vi "Manage sensor alert.vi"(7 "Application path":path, 8 "Error In":errorcluster, 9 "Humidity":dbl, 10 "Temperature":dbl, 11 "MAC address":string) -> (0 "Error Out":errorcluster)   [LabVIEW 2016]
uses:
  <vilib>/Utility/config.llb/Read Key (Boolean).vi
  <vilib>/Utility/config.llb/Read Key (Double).vi
  <vilib>/Utility/config.llb/Read Key (String).vi
  <vilib>/Utility/SMTP/NI_SMTPEmail.lvlib
  <vilib>/Utility/config.llb/NI_LVConfig.lvlib
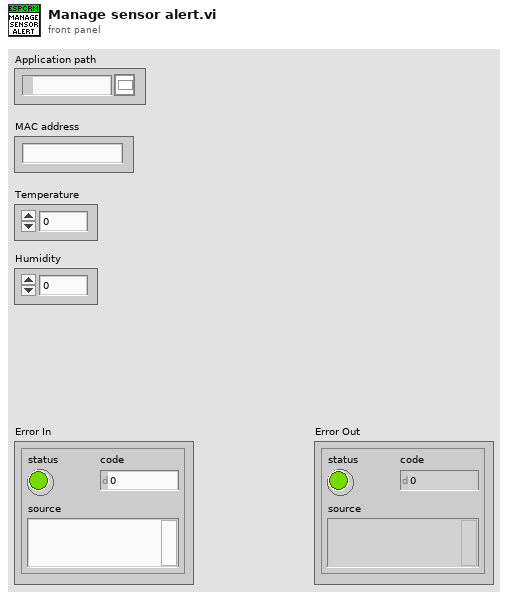
[diagram p1: front panel]
types:
  T1 = typedef "NI_LVConfig.lvlib/Config Data RefNum.ctl" = refnum<k1>
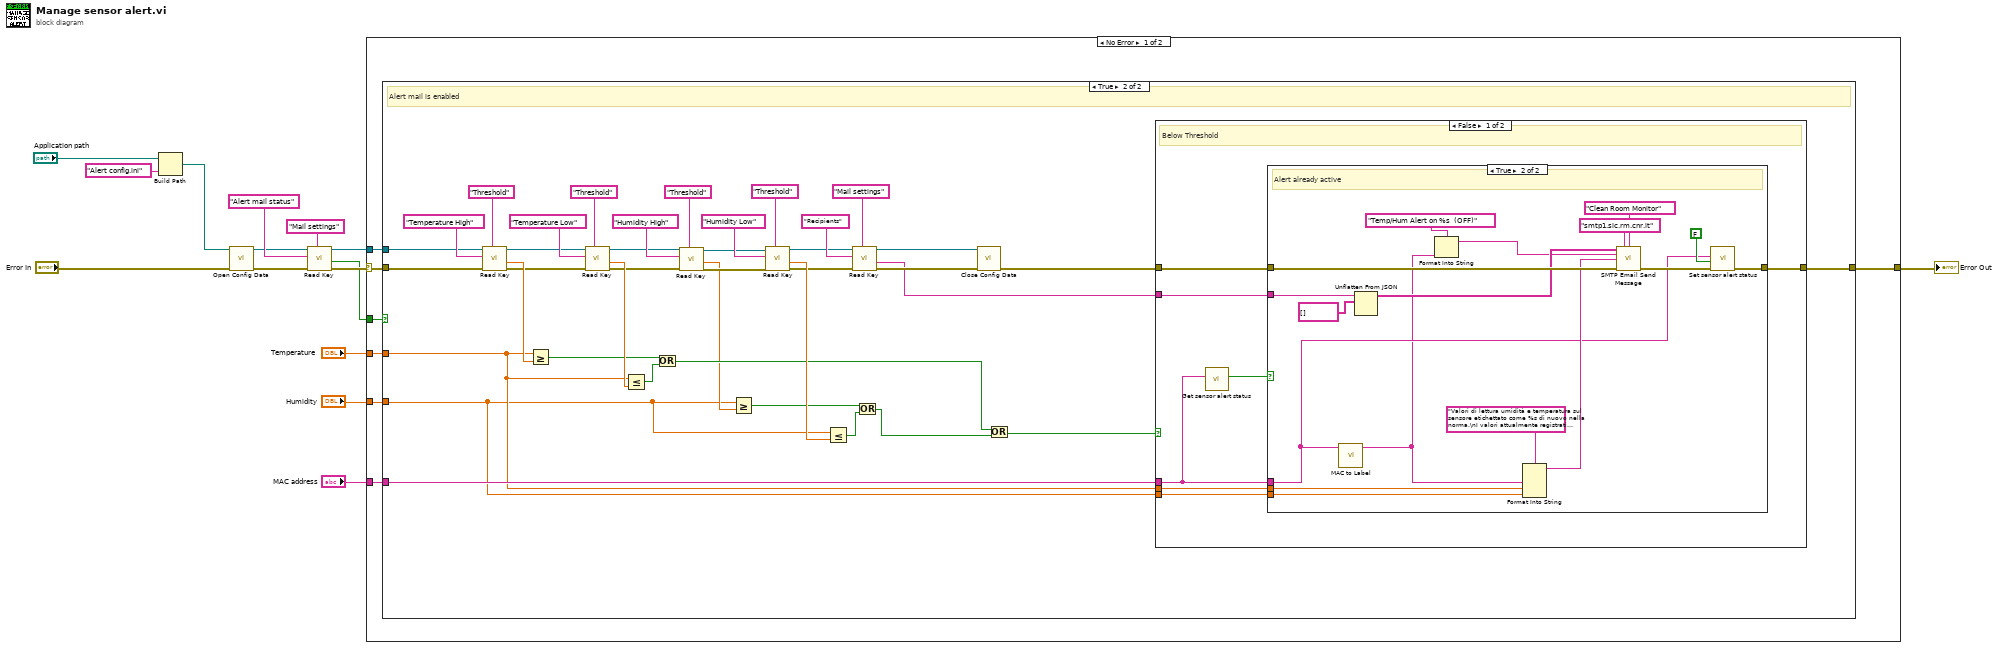
[diagram p0: block diagram]
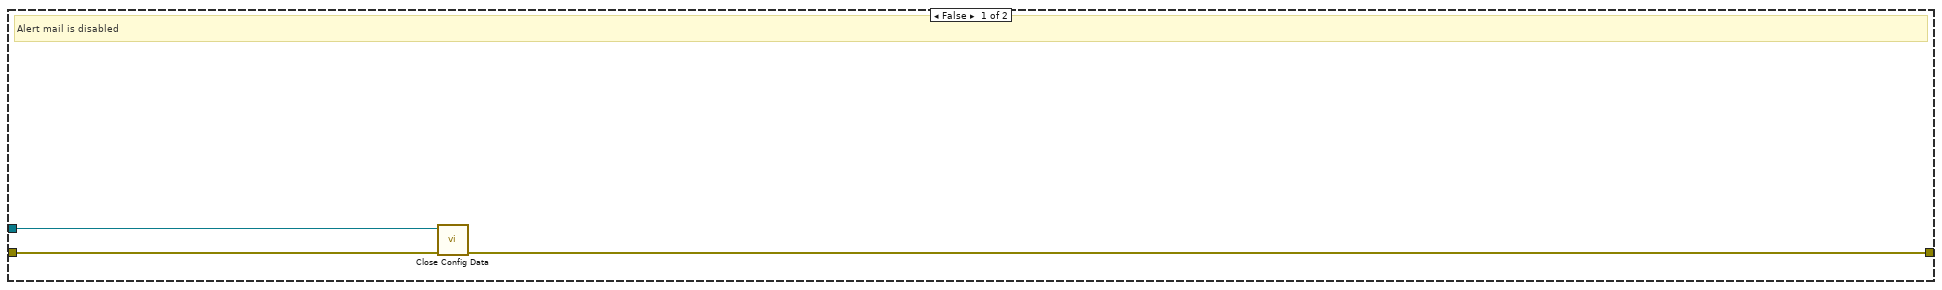
[diagram p2: hidden frame]
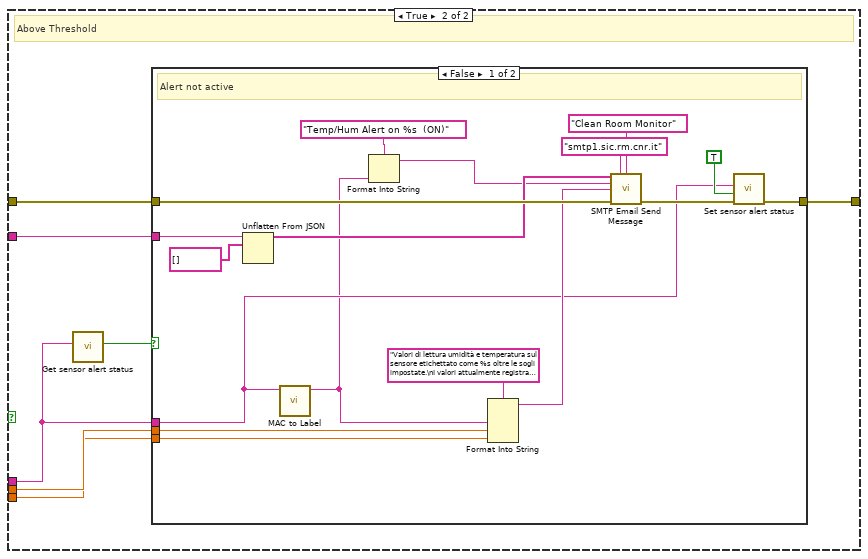
[diagram p4: hidden frame]
diagram:
  n1 = Build Path(base path="Application path", name or relative path="Alert config.ini") -> (appended path=w14:path)
  n2 = call <vilib>:"Open Config Data.vi"("error in (no error)"="Error In", "configuration file path"=w14) -> ("error out"=w9:errorcluster, "refnum"=w10:T1)  [unwired: 7 in, 1 out]
  n3 = call-poly <vilib>:"Read Key.vi"("section"="Mail settings", "error in (no error)"=w9, "key"="Alert mail status", "refnum"=w10) -> ("error out"=w7:errorcluster, "value"=w5:bool, "refnum out"=w8:T1)  [unwired: 4 in, 1 out]
  n4 = case shown="No Error" w7 {
    selector: w7 -> [w21 w115]
    tunnel: [w17 w115] -> w15
    tunnel: w8 -> [w20 _]
    tunnel: w5 -> [w22 _]
    tunnel: "Temperature" -> [w19 _]
    tunnel: "Humidity" -> [w18 _]
    tunnel: "MAC address" -> [w16 _]
    frame No Error {
      n5 = case shown="True" w22 {
        tunnel: w21 -> [w25 w55]
        tunnel: w20 -> [w23 w56]
        tunnel: w19 -> [_ w40]
        tunnel: w18 -> [_ w29]
        tunnel: [w24 w53] -> w17
        tunnel: w16 -> [_ w52]
        frame False {
          # "Alert mail is disabled"
          n6 = call <vilib>:"Close Config Data.vi"("error in (no error)"=w25, "refnum"=w23) -> ("error out"=w24:errorcluster)  [unwired: 8 in, 1 out]
        }
        frame True {
          # "Alert mail is enabled"
          n7 = call-poly <vilib>:"Read Key.vi"("section"="Threshold", "error in (no error)"=w55, "key"="Temperature High", "refnum"=w56) -> ("error out"=w43:errorcluster, "value"=w51:dbl, "refnum out"=w42:T1)  [unwired: 4 in, 1 out]
          n8 = Greater Or Equal?(x=w40, y=w51) -> (x >= y?=w38:bool)
          n9 = call-poly <vilib>:"Read Key.vi"("section"="Threshold", "error in (no error)"=w43, "key"="Temperature Low", "refnum"=w42) -> ("error out"=w33:errorcluster, "value"=w41:dbl, "refnum out"=w34:T1)  [unwired: 4 in, 1 out]
          n10 = Less Or Equal?(x=w40, y=w41) -> (x <= y?=w39:bool)
          n11 = Or(x=w38, y=w39) -> (x .or. y?=w37:bool)
          n12 = call-poly <vilib>:"Read Key.vi"("section"="Threshold", "error in (no error)"=w33, "key"="Humidity High", "refnum"=w34) -> ("error out"=w32:errorcluster, "value"=w30:dbl, "refnum out"=w31:T1)  [unwired: 4 in, 1 out]
          n13 = Greater Or Equal?(x=w29, y=w30) -> (x >= y?=w28:bool)
          n14 = call-poly <vilib>:"Read Key.vi"("section"="Threshold", "error in (no error)"=w32, "key"="Humidity Low", "refnum"=w31) -> ("error out"=w46:errorcluster, "value"=w50:dbl, "refnum out"=w47:T1)  [unwired: 4 in, 1 out]
          n15 = Less Or Equal?(x=w29, y=w50) -> (x <= y?=w27:bool)
          n16 = call-poly <vilib>:"Read Key.vi"("section"="Mail settings", "error in (no error)"=w46, "key"="Recipients", "refnum"=w47) -> ("error out"=w63:errorcluster, "value"=w49:string, "refnum out"=w62:T1)  [unwired: 4 in, 1 out]
          n17 = Or(x=w28, y=w27) -> (x .or. y?=w26:bool)
          n18 = call <vilib>:"Close Config Data.vi"("error in (no error)"=w63, "refnum"=w62) -> ("error out"=w54:errorcluster)  [unwired: 8 in, 1 out]
          n19 = Or(x=w37, y=w26) -> (x .or. y?=w48:bool)
          n20 = case shown="False" w48 {
            tunnel: w54 -> [w70 w96]
            tunnel: [w65 w95] -> w53
            tunnel: w52 -> [w66 w91]
            tunnel: w40 -> [w68 w94]
            tunnel: w29 -> [w67 w93]
            tunnel: w49 -> [w69 w92]
            frame False {
              # "Below Threshold"
              n21 = call "Get sensor alert status.vi"("MAC address"=w66) -> ("Is Alert Active?"=w71:bool)  [unwired: 9 in, 1 out]
              n22 = case shown="True" w71 {
                tunnel: w70 -> [w72 w88]
                tunnel: [w72 w79] -> w65
                tunnel: w66 -> [_ w77]
                tunnel: w68 -> [_ w87]
                tunnel: w67 -> [_ w86]
                tunnel: w69 -> [_ w84]
                frame False {
                  # "Alert not active"
                }
                frame True {
                  # "Alert already active"
                  n23 = call "MAC to Label.vi"("MAC address"=w77) -> ("Label"=w74:string)  [unwired: 9 in, 1 out]
                  n24 = Unflatten From JSON(JSON string=w84, type and defaults=string[] []) -> (value=w82:string[])  [unwired: 5 in, 1 out]
                  n25 = Format Into String(format string="Temp/Hum Alert on %s  (OFF)" ("subject ([No Subject])"), w74) -> (resulting string=w73:string)  [unwired: 2 in, 1 out]
                  n26 = Format Into String(format string="Valori di lettura umidità e temperatura sul sensore etichettato come %s di nuovo nella norma.\nI valori attualmente registrati sono:\nTemperatura: %.1f °C\nUmidità: %.1f %", w74, w87, w86) -> (resulting string=w85:string)  [unwired: 2 in, 1 out]
                  n27 = call <vilib>:"SMTP Email Send Message.vi"("recipients"=w82, "mail server"="smtp1.sic.rm.cnr.it" ("Mail Server 2"), "return address"="Clean Room Monitor", "subject ([No Subject])"=w73, "message"=w85, "error in (no error)"=w88) -> ("error out"=w80:errorcluster)  [unwired: 8 in, 1 out]
                  n28 = call "Set sensor alert status.vi"("Error In"=w80, "Alert status"=FALSE, "MAC address"=w77) -> ("Error Out"=w79:errorcluster)  [unwired: 7 in]
                }
              }
            }
            frame True {
              # "Above Threshold"
              n29 = call "Get sensor alert status.vi"("MAC address"=w91) -> ("Is Alert Active?"=w90:bool)  [unwired: 9 in, 1 out]
              n30 = case shown="False" w90 {
                tunnel: w96 -> [w112 w114]
                tunnel: [w102 w114] -> w95
                tunnel: w91 -> [w100 _]
                tunnel: w94 -> [w110 _]
                tunnel: w93 -> [w109 _]
                tunnel: w92 -> [w107 _]
                frame False {
                  # "Alert not active"
                  n31 = Unflatten From JSON(JSON string=w107, type and defaults=string[] []) -> (value=w105:string[])  [unwired: 5 in, 1 out]
                  n32 = call "MAC to Label.vi"("MAC address"=w100) -> ("Label"=w97:string)  [unwired: 9 in, 1 out]
                  n33 = Format Into String(format string="Temp/Hum Alert on %s  (ON)" ("subject ([No Subject])"), w97) -> (resulting string=w98:string)  [unwired: 2 in, 1 out]
                  n34 = Format Into String(format string="Valori di lettura umidità e temperatura sul sensore etichettato come %s oltre le sogli impostate.\nI valori attualmente registrati sono:\nTemperatura: %.1f °C\nUmidità: %.1f %", w97, w110, w109) -> (resulting string=w108:string)  [unwired: 2 in, 1 out]
                  n35 = call <vilib>:"SMTP Email Send Message.vi"("recipients"=w105, "mail server"="smtp1.sic.rm.cnr.it" ("Mail Server 2"), "return address"="Clean Room Monitor", "subject ([No Subject])"=w98, "message"=w108, "error in (no error)"=w112) -> ("error out"=w103:errorcluster)  [unwired: 8 in, 1 out]
                  n36 = call "Set sensor alert status.vi"("Error In"=w103, "Alert status"=TRUE, "MAC address"=w100) -> ("Error Out"=w102:errorcluster)  [unwired: 7 in]
                }
                frame True {
                  # "Alert already active"
                }
              }
            }
          }
        }
      }
    }
    frame Error {
    }
  }
  "Error Out" <- w15
